vi "SEA-9811_ReceiverAndTransmitter_FPGA_9220_timepulseseeker debug.vi"() -> ()   [LabVIEW 2015]
doc: "This example demonstrates the receiver's functionality. ARINC data can be received with up to 8 channels which can be configured regarding high- or low-speed data rate, label recognition, parity check, decoder functions or label bit order (CONFIG). Up to sixteen 8-bit labels can be stored for label recognition. Duplicate values if you need fewer labels. For more details, look at the RT frontend example.\n\nCopyright (c) 2013 S.E.A. Datentechnik GmbH, Germany"
uses:
  <vilib>/Platform/TimedLoop/XDataNode/timing_clust.ctl
  <vilib>/Platform/TimedLoop/XDataNode/nitl_modes.ctl
  <vilib>/Platform/TimedLoop/XDataNode/wakeup.ctl
  <vilib>/rvi/Emulation/niFpgaGetClockAttributes.vi
  <vilib>/rvi/Emulation/niFpgaSctlEmulationGetInTimedLoop.vi
  <vilib>/rvi/Emulation/niFpgaEmulationReportErrorSimple.vi
  <vilib>/rvi/Emulation/niFpgaCriticalErrorInLSC.vi
  <vilib>/rvi/Emulation/niFpgaProcessEmulError.vi
  <vilib>/rvi/eio/common/nirviEmuTemplateMethod_errors.vi
  GlobalVar.vi
  <vilib>/rvi/eio/common/nirviEmuTemplatePropertyGet_noerrors.vi
  <vilib>/rvi/interface/RandomDataEmulation/niFpgaRandomDataHandleErrors.vi
  <vilib>/rvi/eio/common/nirviEmuTemplatePropertyGet_errors.vi
  <vilib>/Platform/TimedLoop/XDataNode/XDataNode.xnode
  <vilib>/eio/EIONode/EIONode.xnode
  <vilib>/eio/EIOMethodNode/EIOMethodNode.xnode
  <vilib>/eio/EIOPropertyNode/EIOPropertyNode.xnode
  <vilib>/rvi/DataTransferAndStorage/Container/XNode/niFpgaContainer.xnode
  <vilib>/rvi/interface/RandomDataEmulation/nirviRandomDataFpgaReadWriteTemplate.vi
  <vilib>/rvi/eio/common/nirviEmuTemplatePropertySet_errors.vi
  <vilib>/rvi/eio/common/nirviEmuTemplatePropertySet_noerrors.vi
  <userlib>/FPGA Timekeeper 1.1b0/FPGA Timekeeper.lvlib
  <vilib>/Platform/TimedLoop/XDataNode/XDNodeRunTimeDep.lvlib
panel:
  out "RxData 3":u32[](array[numeric])
  out "RxData 2":u32[](array[numeric])
  out "RxData":u32[](array[numeric])
  out "9220_AIs_U32":u32[](array[numeric])
  out "Tx Counter":u32
  out "TxStatus":errorcluster
  out "TxData":errorcluster
  in  "Rx Label Filter":u8[](array[numeric])=[0, 0, 0, 0, 0, 0, 0, 0, 0, 0, 0, 0, 0, 0, 0, 0]
  out "Pulse":bool
  out "Counter":u32
  in  "AI0_threshold (V)":fxp<+/-,24,5>=5.0
  in  "Pulse length (ms)":u32
  in  "FPGA Loop rate (usec)":u16
  out "9220_AIs":fxp<+/-,24,5>[](array[numeric])
  out "Rx rate us":u32
  out "Elements in FIFO":u32
  out "FPGA Timekeeper time (ns)":u64
  out "FPGA Timekeeper locked":bool
  out "offset from RT time (ns)":i32
  in  "RT time (ns)":u64
  in  "Finished config":bool
  in  "Configure\nchannel":bool
  out "Rx Status":u16 format="%016b"
  out "Tx Status":u8 format="%08b"
  in  "Tx Data":u32=305419896 format="%08x"
  in  "Tx Config Data (TCR)":u16=8192 format="%04x"
  in  "Transmit Data":bool
  out "DMA Overflow":bool
  in  "Rx Channel Number":u8 max=7 step=1
  in  "Rx Config Data (RCR)":u16=32 format="%04x"
  # "Please refer to VI description for instructions!"
  # "Receiver Configuration"
  # "DMA Status"
  # "Transmitter"
  # "Order for tags is\n8,9,0,1,2,3,4,5,6,7"
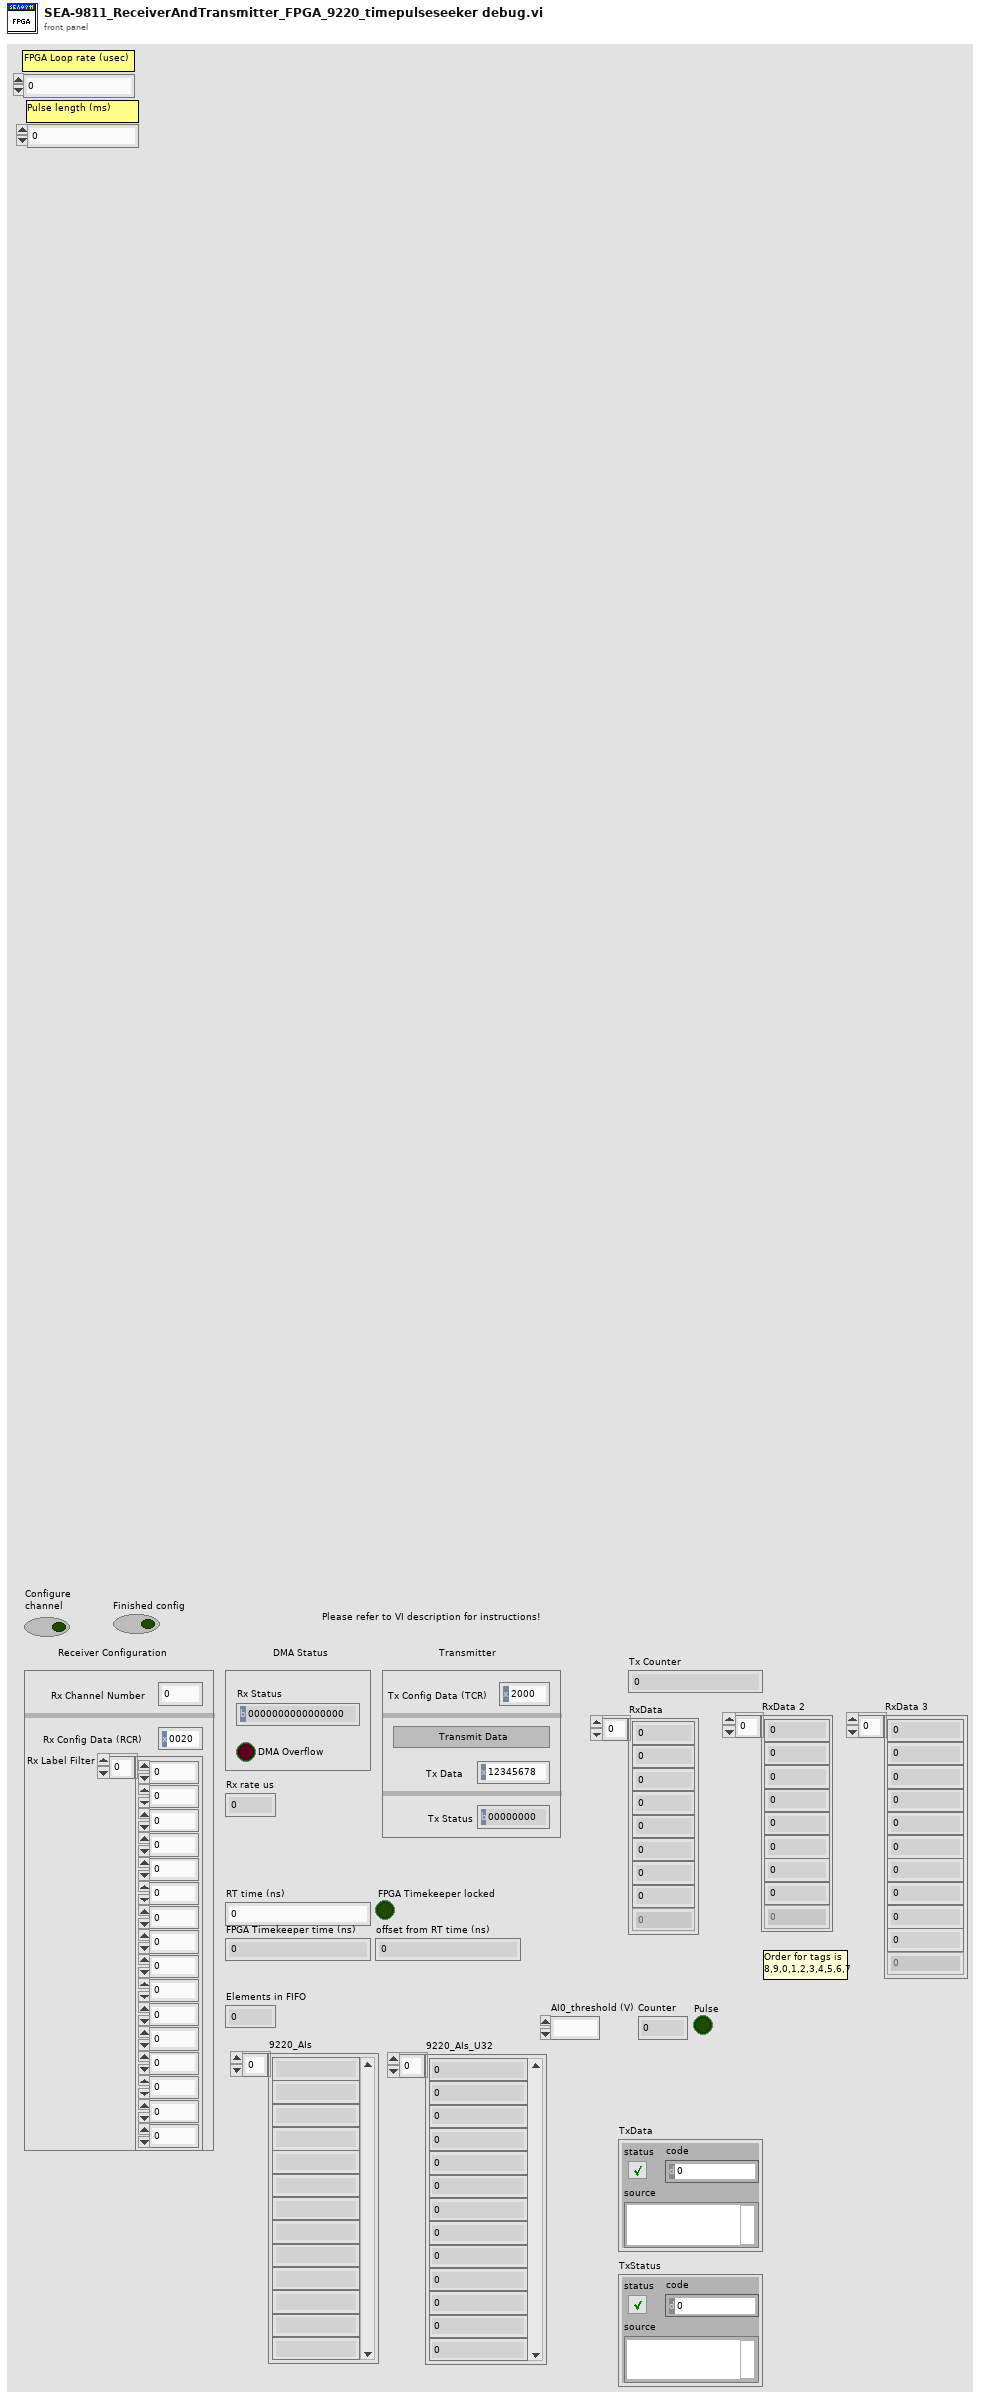
[diagram p1: front panel]
types:
  T1 = cluster{"Rx Label Filter[0]":u8, "Rx Label Filter[1]":u8, "Rx Label Filter[2]":u8, "Rx Label Filter[3]":u8, "Rx Label Filter[4]":u8, "Rx Label Filter[5]":u8, "Rx Label Filter[6]":u8, "Rx Label Filter[7]":u8, "Rx Label Filter[8]":u8, "Rx Label Filter[9]":u8, "Rx Label Filter[10]":u8, "Rx Label Filter[11]":u8, "Rx Label Filter[12]":u8, "Rx Label Filter[13]":u8, "Rx Label Filter[14]":u8, "Rx Label Filter[15]":u8}
  T2 = typedef "XDNodeRunTimeDep.lvlib/timing_clust.ctl" = cluster{"Expected End [f-1]":u64, "Actual End [f-1]":u64, "Finished Late? [f-1]":bool, "Expected End [i-1]":u64, "Actual End [i-1]":u64, "Finished Late? [i-1]":bool, "Expected Start [i]":u64, "Actual Start [i]":u64, "Expected Start [f]":u64, "Actual Start [f]":u64, "Source Name":string, "Structure Name":string, "Period":i64, "Deadline":i64, "Offset":i64, "Start":i64, "Priority":i32, "Timeout":i32, "Mode":T3, "Wakeup Reason":T4, "Error":errorcluster, "Source Type":string, "Secondary Source Type":string, "Global End Time":u64, "Global Start Time":u64, "Frame Duration":u64, "Iteration Duration":u64, "Assigned CPU":i32, "I/O Scan Engine Mode":u32}
  T3 = typedef "XDNodeRunTimeDep.lvlib/nitl_modes.ctl" = enum32{"No Change", "Process missed periods, maintain original phase", "Discard missed periods, maintain original phase", "Process missed periods, ignore original phase", "Discard missed periods, ignore original phase"}
  T4 = typedef "XDNodeRunTimeDep.lvlib/wakeup.ctl" = enum32{"Normal", "Aborted", "Asynchronous wakeup", "Timing source error", "Timed loop error", "Timeout"}
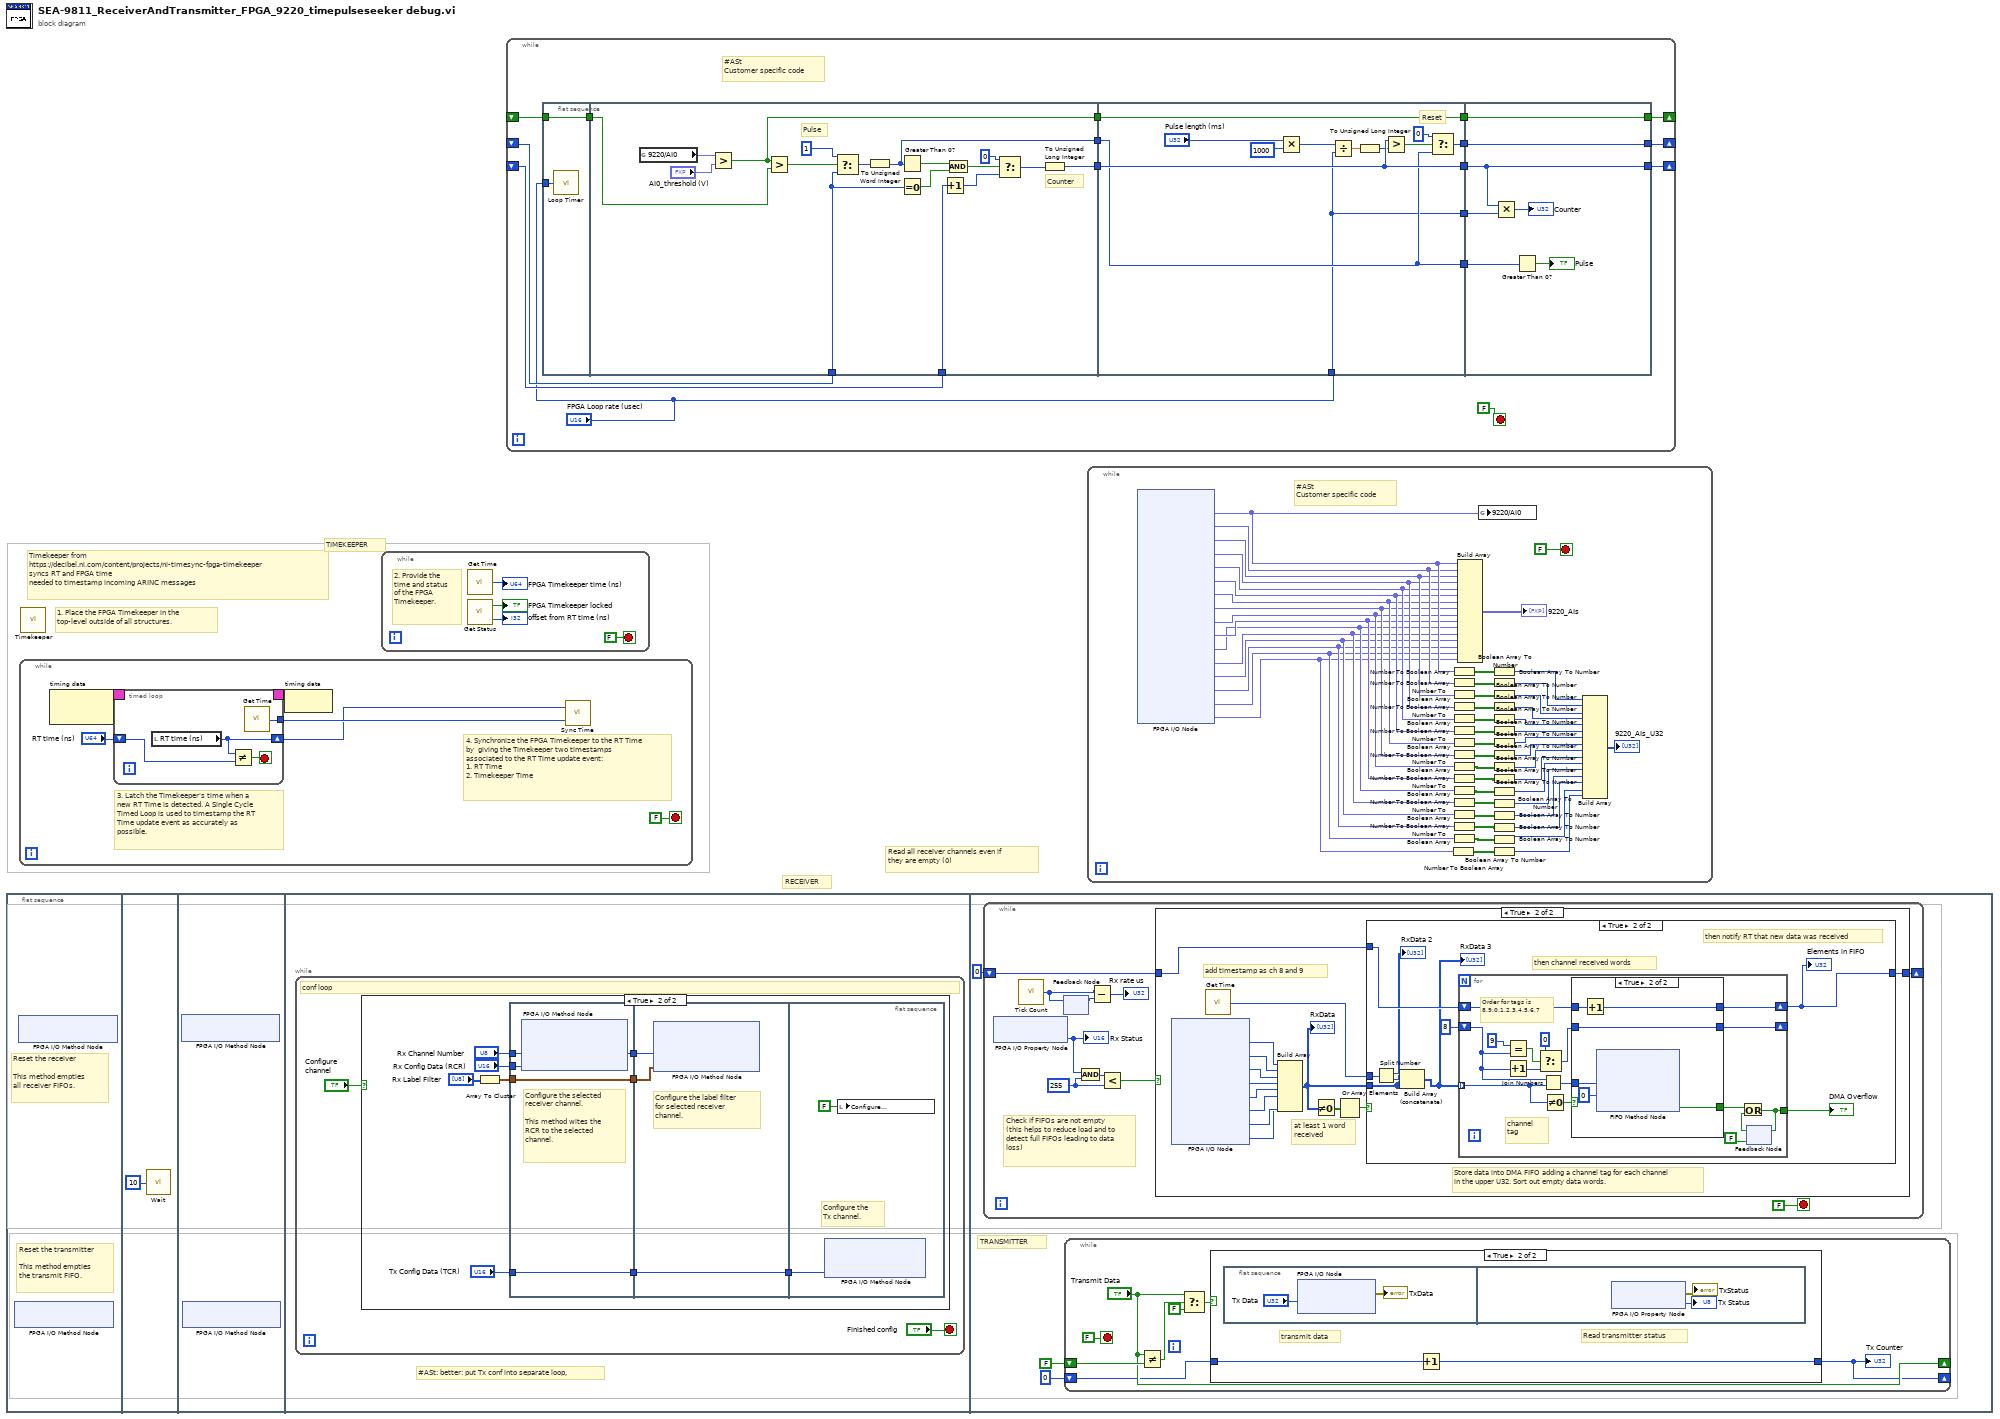
[diagram p0: block diagram]
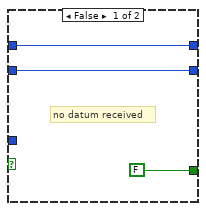
[diagram p6: hidden frame]
diagram:
  # "Read all receiver channels even if they are empty (0)"
  # "TIMEKEEPER"
  # "Timekeeper from\nhttps://decibel.ni.com/content/projects/ni-timesync-fpga-timekeeper\nsyncs RT and FPGA time\nneeded to timestamp incoming ARINC messages"
  # "1. Place the FPGA Timekeeper in the top-level outside of all structures."
  # "RECEIVER"
  n1 = flat-sequence {
    frame #0 {
      # "Reset the transmitter\n\nThis method empties\nthe transmit FIFO."
      # "Reset the receiver\n\nThis method empties\nall receiver FIFOs."
      n2 = xnode "FPGA I/O Method Node"() -> ()  [unwired: 1 in, 1 out]
      n3 = xnode "FPGA I/O Method Node"() -> ()  [unwired: 1 in, 1 out]
    }
    frame #1 {
      n4 = call "Wait"("Count(mSec)"=u32 10) -> ()  [unwired: 1 out]
    }
    frame #2 {
      n5 = xnode "FPGA I/O Method Node"() -> ()  [unwired: 1 in, 1 out]
      n6 = xnode "FPGA I/O Method Node"() -> ()  [unwired: 1 in, 1 out]
    }
    frame #3 {
      # "#ASt: better: put Tx conf into separate loop,"
      n7 = while {
        stop <- "Finished config" stop-if-true
        # "conf loop"
        n8 = case shown="True" "Configure\nchannel" {
          frame False {
          }
          frame True {
            n9 = Array To Cluster(array="Rx Label Filter") -> (cluster=w4:T1)
            n10 = flat-sequence {
              tunnel: "Rx Channel Number" -> [w16]
              tunnel: [w16] -> w12
              tunnel: "Rx Config Data (RCR)" -> [w15]
              tunnel: [w14] -> w11
              tunnel: w4 -> [w14]
              tunnel: "Tx Config Data (TCR)" -> [w13]
              tunnel: [w13] -> w6
              tunnel: w12 -> [w19]
              tunnel: w11 -> [w18]
              tunnel: [w17] -> w7
              tunnel: w6 -> [w17]
              tunnel: w7 -> [w21]
              frame #0 {
                # "Configure the selected\nreceiver channel.\n\nThis method wites the\nRCR to the selected\nchannel."
                n11 = xnode "FPGA I/O Method Node"("Channel Number"=w16, "Control Register"=w15) -> ()  [unwired: 1 in, 1 out]
              }
              frame #1 {
                # "Configure the label filter\nfor selected receiver\nchannel."
                n12 = xnode "FPGA I/O Method Node"("Channel Number"=w19, "Label Filter"=w18) -> ()  [unwired: 1 in, 1 out]
              }
              frame #2 {
                # "Configure the\nTx channel."
                n13 = xnode "FPGA I/O Method Node"("Control Register"=w21) -> ()  [unwired: 1 in, 1 out]
                n14 = local write "Configure\nchannel"(FALSE ("Configure\nchannel")) -> ()
              }
            }
          }
        }
      }
    }
    frame #4 {
      # "TRANSMITTER"
      n15 = while {
        shift-right: [w43] -> _
        shift-left: u32 0 -> [w44]
        stop <- FALSE stop-if-true
        w46 = u16 255 ("y")
        # "Check if FIFOs are not empty\n(this helps to reduce load and to detect full FIFOs leading to data loss)"
        n16 = xnode "FPGA I/O Property Node"() -> ("Rx Status"=w48:u16)  [unwired: 1 in, 1 out]
        "Rx Status" <- w48
        n17 = call "Tick Count"() -> ("Tick Count(uSec)"=w42:u32)
        n18 = feedback-in #1(w42) -> ()
        n19 = feedback #1() -> (w41:u32)  [unwired: 1 in]
        n20 = And(x=w48, y=w46) -> (x .and. y?=w47:u16)
        n21 = Subtract(x=w42, y=w41) -> (x-y=→"Rx rate us":u32)
        n22 = Less?(x=w47, y=w46) -> (x < y?=w45:bool)
        n23 = case shown="True" w45 {
          tunnel: w44 -> [w50 w56]
          tunnel: [w50 w55] -> w43
          frame False {
          }
          frame True {
            # "add timestamp as ch 8 and 9"
            # "at least 1 word\nreceived"
            # "Store data into DMA FIFO adding a channel tag for each channel in the upper U32. Sort out empty data words."
            n24 = xnode "FPGA I/O Node"() -> ("Mod1/Rx0"=w58:u32, "Mod1/Rx1"=w59:u32, "Mod1/Rx2"=w60:u32, "Mod1/Rx3"=w61:u32, "Mod1/Rx4"=w62:u32, "Mod1/Rx5"=w63:u32, "Mod1/Rx6"=w64:u32, "Mod1/Rx7"=w57:u32)  [unwired: 8 in, 8 out]
            n25 = call <userlib>:"Get Time.vi"() -> ("time (ns)"=w51:u64)
            n26 = Build Array(w58, w59, w60, w61, w62, w63, w64, w57) -> (w54:u32[])
            "RxData" <- w54
            n27 = Not Equal To 0?(x=w54) -> (x != 0?=w53:bool[])
            n28 = Or Array Elements(Boolean array=w53) -> (logical OR=w52:bool)
            n29 = case shown="True" w52 {
              tunnel: w56 -> [w65 w68]
              tunnel: [w65 w74] -> w55
              tunnel: w54 -> [_ w67]
              tunnel: w51 -> [_ w69]
              frame False {
              }
              frame True {
                # "then notify RT that new data was received"
                # "then channel received words"
                n30 = Split Number(x=w69) -> (hi(x)=w71:u32, lo(x)=w70:u32)
                n31 = Build Array (concatenate)(w71, w70, w67) -> (w66:u32[])
                "RxData 3" <- w66
                n32 = for {
                  tunnel: w66 -> [w82] mode=indexing
                  tunnel: [w87] -> w73
                  shift-right: [w83] -> w74
                  shift-left: w68 -> [w84]
                  shift-right: [w75] -> _
                  shift-left: u32 8 ("hi") -> [w79]
                  # "Order for tags is\n8,9,0,1,2,3,4,5,6,7"
                  # "channel\ntag"
                  n33 = Equal?(x=u32 9, y=w79) -> (x = y?=w80:bool)
                  n34 = Increment(x=w79) -> (x+1=w81:u32)
                  n35 = Select(t=u32 0, s=w80, f=w81) -> (s? t:f=w76:u32)
                  n36 = Join Numbers(hi=w79, lo=w82) -> ((hi.lo)=w85:u64)
                  n37 = Not Equal To 0?(x=w82) -> (x != 0?=w86:bool)
                  n38 = case shown="True" w86 {
                    tunnel: [FALSE ("Timed Out?") w99] -> w88
                    tunnel: w85 -> [_ w96]
                    tunnel: w84 -> [w92 w98]
                    tunnel: [w92 w97] -> w83
                    tunnel: w76 -> [w91 w94]
                    tunnel: [w91 w94] -> w75
                    frame False {
                      # "no datum received"
                    }
                    frame True {
                      n39 = Increment(x=w98) -> (x+1=w97:u32)
                      n40 = xnode ("FIFO Method Node")("Element"=w96, "Timeout"=0) -> ("Timed Out?"=w99:bool)  [unwired: 1 in, 1 out]
                    }
                  }
                  n41 = feedback #2(FALSE) -> (w89:bool)
                  n42 = Or(x=w88, y=w89) -> (x .or. y?=w87:bool)
                  n43 = feedback-in #2(w87) -> ()
                }
                "DMA Overflow" <- w73
                "Elements in FIFO" <- w74
                "RxData 2" <- w67
              }
            }
          }
        }
      }
      n44 = while {
        shift-right: ["Transmit Data"] -> _
        shift-left: FALSE ("Transmit Data") -> [w31]
        shift-right: [w26] -> _
        shift-left: u32 0 ("Tx Counter") -> [w25]
        stop <- FALSE stop-if-true
        n45 = Not Equal?(x="Transmit Data", y=w31) -> (x != y?=w29:bool)
        n46 = Select(t="Transmit Data", s=w29, f=FALSE) -> (s? t:f=w30:bool)
        n47 = case shown="True" w30 {
          tunnel: [w33 w34] -> w26
          tunnel: w25 -> [w33 w35]
          frame False {
          }
          frame True {
            # "Read transmitter status"
            # "transmit data"
            n48 = flat-sequence {
              frame #0 {
                n49 = xnode "FPGA I/O Node"("Mod1/Tx0"="Tx Data") -> ("error out"=→"TxData":errorcluster)  [unwired: 2 in, 1 out]
              }
              frame #1 {
                n50 = xnode "FPGA I/O Property Node"() -> ("error out"=→"TxStatus":errorcluster, "Tx Status"=→"Tx Status":u8)  [unwired: 2 in, 1 out]
              }
            }
            n51 = Increment(x=w35) -> (x+1=w34:u32)
          }
        }
        "Tx Counter" <- w26
      }
    }
  }
  n52 = while {
    stop <- FALSE stop-if-true
    # "3. Latch the Timekeeper's time when a new RT Time is detected. A Single Cycle Timed Loop is used to timestamp the RT Time update event as accurately as possible."
    # "4. Synchronize the FPGA Timekeeper to the RT Time by  giving the Timekeeper two timestamps associated to the RT Time update event:\n1. RT Time\n2. Timekeeper Time"
    n53 = node-c288() -> (w105:T2)  [unwired: 1 in]
    n54 = timed-loop {
      timing: w105 -> [_]
      timing-out: [_] -> w104
      shift-right: [w106] -> w100
      shift-left: "RT time (ns)" -> [w107]
      tunnel: [w109] -> w103
      stop <- w108 stop-if-true
      n55 = local read "RT time (ns)"() -> (w106:u64)
      n56 = Not Equal?(x=w106, y=w107) -> (x != y?=w108:bool)
      n57 = call <userlib>:"Get Time.vi"() -> ("time (ns)"=w109:u64)
    }
    n58 = node-c288(w104) -> ()
    n59 = call <userlib>:"Sync Time.vi"("FPGA Timekeeper time (ns)"=w103, "time reference time (ns)"=w100) -> ()
  }
  n60 = call <userlib>:"Timekeeper.vi"() -> ()  [unwired: 12 in]
  n61 = while {
    stop <- FALSE stop-if-true
    # "2. Provide the time and status of the FPGA Timekeeper."
    n62 = call <userlib>:"Get Time.vi"() -> ("time (ns)"=→"FPGA Timekeeper time (ns)":u64)
    n63 = call <userlib>:"Get Status.vi"() -> ("FPGA Timekeeper locked"=→"FPGA Timekeeper locked":bool, "offset from time reference"=→"offset from RT time (ns)":i32)
  }
  n64 = while {
    shift-right: [w133] -> _
    shift-left: _ -> [w132]
    shift-right: [w131] -> _
    shift-left: _ -> [w126]
    shift-right: [w127] -> _
    shift-left: _ -> [w125]
    stop <- FALSE stop-if-true
    # "#ASt\nCustomer specific code"
    n65 = flat-sequence {
      tunnel: w132 -> [w136]
      tunnel: [w136] -> w124
      tunnel: "FPGA Loop rate (usec)" -> [w135]
      tunnel: [w137] -> w130
      tunnel: [w141] -> w129
      tunnel: [w140] -> w128
      tunnel: w126 -> [w144]
      tunnel: w125 -> [w143]
      tunnel: w124 -> [w153]
      tunnel: w128 -> [w161]
      tunnel: w129 -> [w155]
      tunnel: w130 -> [w165]
      tunnel: "FPGA Loop rate (usec)" -> [w154]
      tunnel: [w165] -> w122
      tunnel: [w164] -> w121
      tunnel: [w161] -> w120
      tunnel: [w155] -> w119
      tunnel: [w154] -> w118
      tunnel: [w169] -> w127
      tunnel: [w171] -> w131
      tunnel: [w172] -> w133
      tunnel: w122 -> [w172]
      tunnel: w121 -> [w171]
      tunnel: w120 -> [w169]
      tunnel: w119 -> [w170]
      tunnel: w118 -> [w168]
      frame #0 {
        n66 = call "Loop Timer"("Count(uSec)"=w135) -> ()  [unwired: 1 out]
      }
      frame #1 {
        # "Pulse"
        # "Counter"
        n67 = global read "GlobalVar.vi" "9220/AI0"() -> (w139:fxp<+/-,24,5>)
        n68 = Greater?(x=w139, y="AI0_threshold (V)") -> (0:w137:bool)
        n69 = Greater?(x=w137, y=w153) -> (0:w152:bool)
        n70 = Select(t=u8 1, s=w152, f=w144) -> (s? t:f=w150:u16)
        n71 = To Unsigned Word Integer(number=w150) -> (unsigned 16bit integer=w141:u16)
        n72 = Greater Than 0?(x=w141) -> (x > 0?=w149:bool)
        n73 = Equal To 0?(x=w144) -> (x = 0?=w148:bool)
        n74 = Increment(x=w143) -> (x+1=w145:u32)
        n75 = And(x=w149, y=w148) -> (x .and. y?=w147:bool)
        n76 = Select(t=u8 0, s=w147, f=w145) -> (s? t:f=w142:u32)
        n77 = To Unsigned Long Integer(number=w142) -> (unsigned 32bit integer=w140:u32)
      }
      frame #2 {
        # "Reset"
        n78 = Multiply(x="Pulse length (ms)", y=i16 1000) -> (x*y=w158:u32)
        n79 = Divide(x=w158, y=w154) -> (x/y=w156:sgl)
        n80 = To Unsigned Long Integer(number=w156) -> (unsigned 32bit integer=w157:u32)
        n81 = Greater?(x=w161, y=w157) -> (0:w162:bool)
        n82 = Select(t=u8 0, s=w162, f=w155) -> (s? t:f=w164:u16)
      }
      frame #3 {
        n83 = Multiply(x=w169, y=w168) -> (x*y=→"Counter":u32)
        n84 = Greater Than 0?(x=w170) -> (x > 0?=→"Pulse":bool)
      }
    }
  }
  n85 = while {
    stop <- FALSE stop-if-true
    # "#ASt\nCustomer specific code"
    n86 = xnode "FPGA I/O Node"() -> ("9220/AI0"=w221:fxp<+/-,24,5>, "9220/AI1"=w220:fxp<+/-,24,5>, "9220/AI2"=w219:fxp<+/-,24,5>, "9220/AI3"=w218:fxp<+/-,24,5>, "9220/AI4"=w217:fxp<+/-,24,5>, "9220/AI5"=w211:fxp<+/-,24,5>, "9220/AI6"=w210:fxp<+/-,24,5>, "9220/AI7"=w209:fxp<+/-,24,5>, "9220/AI8"=w208:fxp<+/-,24,5>, "9220/AI9"=w207:fxp<+/-,24,5>, "9220/AI10"=w206:fxp<+/-,24,5>, "9220/AI11"=w205:fxp<+/-,24,5>, "9220/AI12"=w204:fxp<+/-,24,5>, "9220/AI13"=w203:fxp<+/-,24,5>, "9220/AI14"=w202:fxp<+/-,24,5>, "9220/AI15"=w201:fxp<+/-,24,5>)  [unwired: 16 in, 16 out]
    n87 = Number To Boolean Array(number=w201) -> (Boolean array=w190:bool[])
    n88 = Number To Boolean Array(number=w221) -> (Boolean array=w216:bool[])
    n89 = Number To Boolean Array(number=w220) -> (Boolean array=w215:bool[])
    n90 = Number To Boolean Array(number=w219) -> (Boolean array=w214:bool[])
    n91 = Number To Boolean Array(number=w218) -> (Boolean array=w213:bool[])
    n92 = Number To Boolean Array(number=w217) -> (Boolean array=w212:bool[])
    n93 = Number To Boolean Array(number=w211) -> (Boolean array=w200:bool[])
    n94 = Number To Boolean Array(number=w210) -> (Boolean array=w199:bool[])
    n95 = Number To Boolean Array(number=w209) -> (Boolean array=w198:bool[])
    n96 = Number To Boolean Array(number=w208) -> (Boolean array=w197:bool[])
    n97 = Number To Boolean Array(number=w207) -> (Boolean array=w196:bool[])
    n98 = Number To Boolean Array(number=w206) -> (Boolean array=w195:bool[])
    n99 = Number To Boolean Array(number=w205) -> (Boolean array=w194:bool[])
    n100 = Number To Boolean Array(number=w204) -> (Boolean array=w193:bool[])
    n101 = Number To Boolean Array(number=w203) -> (Boolean array=w192:bool[])
    n102 = Number To Boolean Array(number=w202) -> (Boolean array=w191:bool[])
    n103 = Build Array(w221, w220, w219, w218, w217, w211, w210, w209, w208, w207, w206, w205, w204, w203, w202, w201) -> (→"9220_AIs":fxp<+/-,24,5>[])
    n104 = global write "GlobalVar.vi" "9220/AI0"(w221) -> ()
    n105 = Boolean Array To Number(Boolean array=w216) -> (number=w189:u32)
    n106 = Boolean Array To Number(Boolean array=w215) -> (number=w188:u32)
    n107 = Boolean Array To Number(Boolean array=w214) -> (number=w187:u32)
    n108 = Boolean Array To Number(Boolean array=w213) -> (number=w186:u32)
    n109 = Boolean Array To Number(Boolean array=w212) -> (number=w185:u32)
    n110 = Boolean Array To Number(Boolean array=w200) -> (number=w184:u32)
    n111 = Boolean Array To Number(Boolean array=w199) -> (number=w183:u32)
    n112 = Boolean Array To Number(Boolean array=w198) -> (number=w182:u32)
    n113 = Boolean Array To Number(Boolean array=w197) -> (number=w181:u32)
    n114 = Boolean Array To Number(Boolean array=w196) -> (number=w180:u32)
    n115 = Boolean Array To Number(Boolean array=w195) -> (number=w179:u32)
    n116 = Boolean Array To Number(Boolean array=w194) -> (number=w178:u32)
    n117 = Boolean Array To Number(Boolean array=w193) -> (number=w177:u32)
    n118 = Boolean Array To Number(Boolean array=w192) -> (number=w176:u32)
    n119 = Boolean Array To Number(Boolean array=w191) -> (number=w175:u32)
    n120 = Boolean Array To Number(Boolean array=w190) -> (number=w174:u32)
    n121 = Build Array(w189, w188, w187, w186, w185, w184, w183, w182, w181, w180, w179, w178, w177, w176, w175, w174) -> (→"9220_AIs_U32":u32[])
  }
